vi "ParamsRuido.vi"(2 "paramsIn":variant) -> (16 "paramsOut":variant)   [LabVIEW 2017]
uses:
  Typedefs/Tipo_ParamsRuido.ctl
panel:
  in  "Init":bool
  in  "Freq. Superior (Hz)":dbl
  in  "Freq. Inferior (Hz)":dbl
  in  "Banda":bool
  in  "Amplitude":dbl
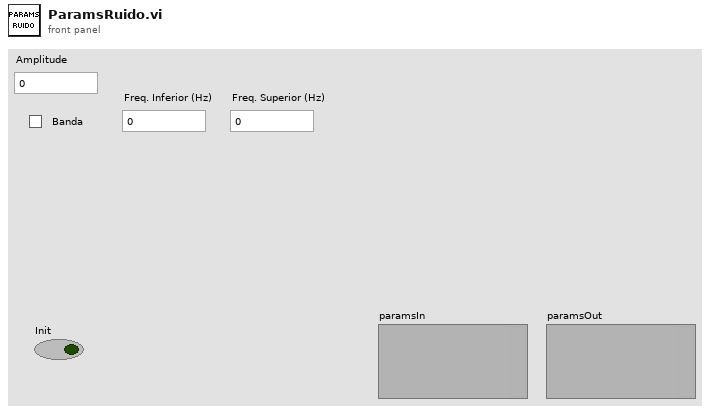
[diagram p1: front panel]
types:
  T1 = typedef "Tipo_ParamsRuido.ctl" = cluster{"Amplitude":dbl, "Banda: ":bool, "Freq. Inferior":dbl, "Freq. Superior":dbl}
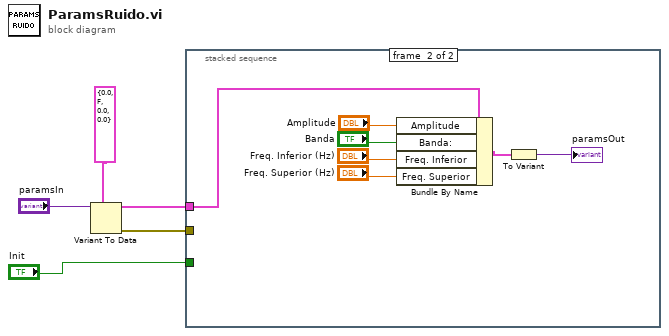
[diagram p0: block diagram]
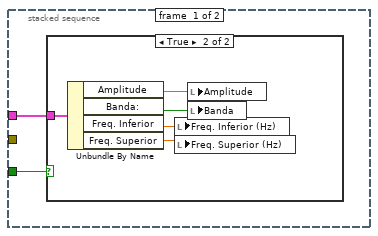
[diagram p2: hidden frame]
diagram:
  n1 = Variant To Data(type=T1 {"Amplitude"=0.0, "Banda: "=FALSE, "Freq. Inferior"=0.0, "Freq. Superior"=0.0} ("ParamsIn"), Variant="paramsIn") -> (data=w3:T1, error out=w1:errorcluster)  [unwired: 1 in]
  n2 = stacked-sequence {
    tunnel: w3 -> [w7 w19]
    tunnel: "Init" -> [w6 _]
    tunnel: w1 -> [_ _]
    frame #0 {
      n3 = case shown="True" w6 {
        tunnel: w7 -> [_ w12]
        frame False {
        }
        frame True {
          n4 = Unbundle By Name(w12) -> ("Amplitude"=w11:dbl, "Banda:"=w10:bool, "Freq. Inferior"=w9:dbl, "Freq. Superior"=w8:dbl)
          n5 = local write "Freq. Inferior (Hz)"(w9) -> ()
          n6 = local write "Freq. Superior (Hz)"(w8) -> ()
          n7 = local write "Amplitude"(w11) -> ()
          n8 = local write "Banda"(w10) -> ()
        }
      }
    }
    frame #1 {
      n9 = Bundle By Name(cluster=w19, "Amplitude"="Amplitude", "Banda:"="Banda", "Freq. Inferior"="Freq. Inferior (Hz)", "Freq. Superior"="Freq. Superior (Hz)") -> (w14:T1)
      n10 = To Variant(anything=w14) -> (Variant=→"paramsOut":variant)
    }
  }
